vi "Trio - Lookup Axis Error.vi"(1 "Error Code":dbl) -> (0 "Error Description":errorcluster)   [LabVIEW 2020, in "TrioMotion Controller.lvlib"]
uses:
  TrioMotion Controller.lvlib
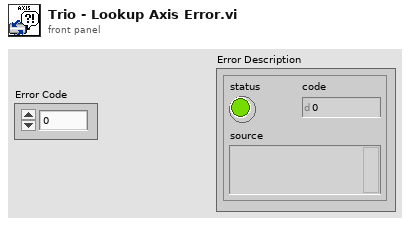
[diagram p1: front panel]
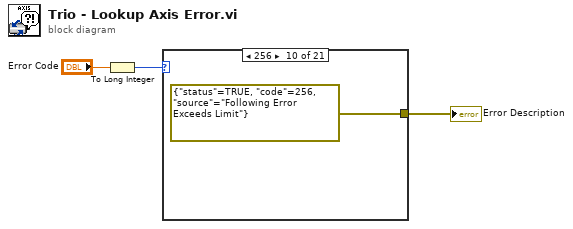
[diagram p0: block diagram]
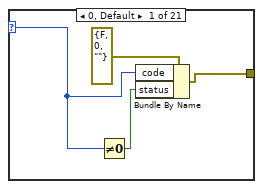
[diagram p2: hidden frame]
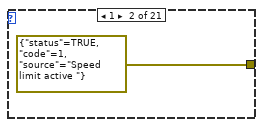
[diagram p3: hidden frame]
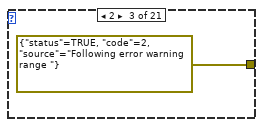
[diagram p4: hidden frame]
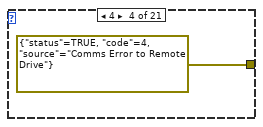
[diagram p5: hidden frame]
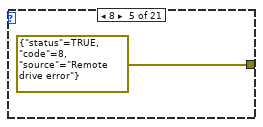
[diagram p6: hidden frame]
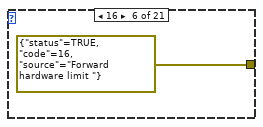
[diagram p7: hidden frame]
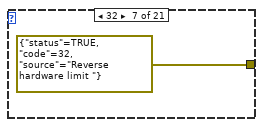
[diagram p8: hidden frame]
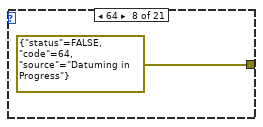
[diagram p9: hidden frame]
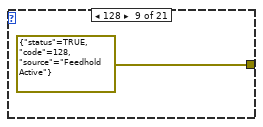
[diagram p10: hidden frame]
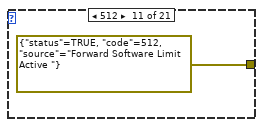
[diagram p11: hidden frame]
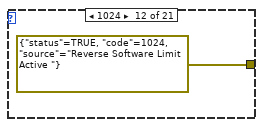
[diagram p12: hidden frame]
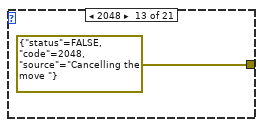
[diagram p13: hidden frame]
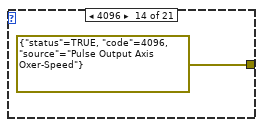
[diagram p14: hidden frame]
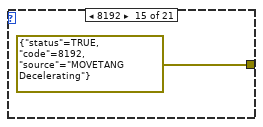
[diagram p15: hidden frame]
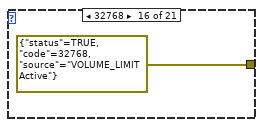
[diagram p16: hidden frame]
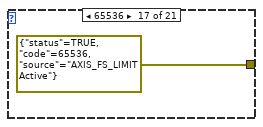
[diagram p17: hidden frame]
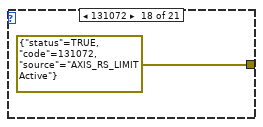
[diagram p18: hidden frame]
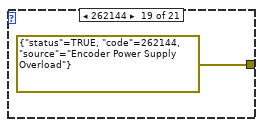
[diagram p19: hidden frame]
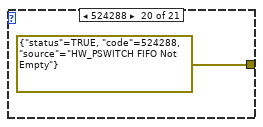
[diagram p20: hidden frame]
diagram:
  n1 = To Long Integer(number="Error Code") -> (32bit integer=w2:i32)
  n2 = case shown="256" w2 {
    selector: w2 -> [w4 _ _ _ _ _ _ _ _ _ _ _ _ _ _ _ _ _ _ _ _]
    tunnel: [w6 errorcluster {"status"=TRUE, "code"=1, "source"="Speed limit active "} ("error in (no error)") errorcluster {"status"=TRUE, "code"=2, "source"="Following error warning range "} ("error in (no error)") errorcluster {"status"=TRUE, "code"=4, "source"="Comms Error to Remote Drive"} ("error in (no error)") errorcluster {"status"=TRUE, "code"=8, "source"="Remote drive error"} ("error in (no error)") errorcluster {"status"=TRUE, "code"=16, "source"="Forward hardware limit "} ("error in (no error)") errorcluster {"status"=TRUE, "code"=32, "source"="Reverse hardware limit "} ("error in (no error)") errorcluster {"status"=FALSE, "code"=64, "source"="Datuming in Progress"} ("error in (no error)") errorcluster {"status"=TRUE, "code"=128, "source"="Feedhold Active"} ("error in (no error)") errorcluster {"status"=TRUE, "code"=256, "source"="Following Error Exceeds Limit"} ("error in (no error)") errorcluster {"status"=TRUE, "code"=512, "source"="Forward Software Limit Active "} ("error in (no error)") errorcluster {"status"=TRUE, "code"=1024, "source"="Reverse Software Limit Active "} ("error in (no error)") errorcluster {"status"=FALSE, "code"=2048, "source"="Cancelling the move "} ("error in (no error)") errorcluster {"status"=TRUE, "code"=4096, "source"="Pulse Output Axis Oxer-Speed"} ("error in (no error)") errorcluster {"status"=TRUE, "code"=8192, "source"="MOVETANG Decelerating"} ("error in (no error)") errorcluster {"status"=TRUE, "code"=32768, "source"="VOLUME_LIMIT Active"} ("error in (no error)") errorcluster {"status"=TRUE, "code"=65536, "source"="AXIS_FS_LIMIT Active"} ("error in (no error)") errorcluster {"status"=TRUE, "code"=131072, "source"="AXIS_RS_LIMIT Active"} ("error in (no error)") errorcluster {"status"=TRUE, "code"=262144, "source"="Encoder Power Supply Overload"} ("error in (no error)") errorcluster {"status"=TRUE, "code"=524288, "source"="HW_PSWITCH FIFO Not Empty"} ("error in (no error)") errorcluster {"status"=TRUE, "code"=1048576, "source"="HW_PSWITCH FIFO Full"} ("error in (no error)")] -> w3
    frame 0, Default {
      n3 = Not Equal To 0?(x=w4) -> (x != 0?=w5:bool)
      n4 = Bundle By Name(cluster=errorcluster {"status"=FALSE, "code"=0, "source"=""} ("error in (no error)"), "code"=w4, "status"=w5) -> (w6:errorcluster)
    }
    frame 1 {
    }
    frame 2 {
    }
    frame 4 {
    }
    frame 8 {
    }
    frame 16 {
    }
    frame 32 {
    }
    frame 64 {
    }
    frame 128 {
    }
    frame 256 {
    }
    frame 512 {
    }
    frame 1024 {
    }
    frame 2048 {
    }
    frame 4096 {
    }
    frame 8192 {
    }
    frame 32768 {
    }
    frame 65536 {
    }
    frame 131072 {
    }
    frame 262144 {
    }
    frame 524288 {
    }
    frame 1048576 {
    }
  }
  "Error Description" <- w3
